vi "Actor Core.vi"(8 "error in":errorcluster, 11 "Assert Startup UI in":refnum<class "Assert Startup UI.lvclass">) -> (0 "error out":errorcluster, 3 "Actor out":refnum<class "Actor.lvclass">)   [LabVIEW 2016, in "Assert Startup UI.lvlib" / "Assert Startup UI.lvclass"]
doc: "(<B>Filename</B>: Actor Framework.lvlib:Actor.lvclass:Actor Core.vi)\n\nReceives messages to the actor, reacts to them, and initiates any error handling that may shut the actor down.\n\nDescendant classes may override this VI to append parallel tasks for the actor to complete while it handles messages. Overrides use the Call Parent Method node."
uses:
  Assert Startup UI.lvclass
  C:/Program Files (x86)/National Instruments/LabVIEW 2016/vi.lib/ActorFramework/Actor/Actor.lvclass
  D:/Work/Projects/Actor_Assert_API/Base UI Actor/Base UI Actor/Base UI Actor.lvclass
  <vilib>/ActorFramework/Actor/Actor.lvclass
  <vilib>/ActorFramework/Message Enqueuer/Message Enqueuer.lvclass
  Assert Startup UI.lvclass/Assert Startup UI.ctl
  Base UI Actor/Base UI Actor/Base UI Actor.lvclass/Base UI Actor.ctl
  <vilib>/ActorFramework/Actor/Actor.lvclass/Actor.ctl
  <vilib>/ActorFramework/Message Enqueuer/Message Enqueuer.lvclass/Message Enqueuer.ctl
  <vilib>/ActorFramework/Message Enqueuer/Init from Existing Queue.vi
  <vilib>/ActorFramework/Message Enqueuer/Enqueue.vi
  <vilib>/ActorFramework/Stop Msg/Stop Msg.lvclass
  C:/Program Files (x86)/National Instruments/LabVIEW 2016/vi.lib/ActorFramework/Message/Message.lvclass
  <vilib>/ActorFramework/Message Priority Queue/Priority Enqueue.vi
  Base UI Actor/Base UI Actor/Base UI Actor.lvclass
panel:
  in  "Add Display":bool
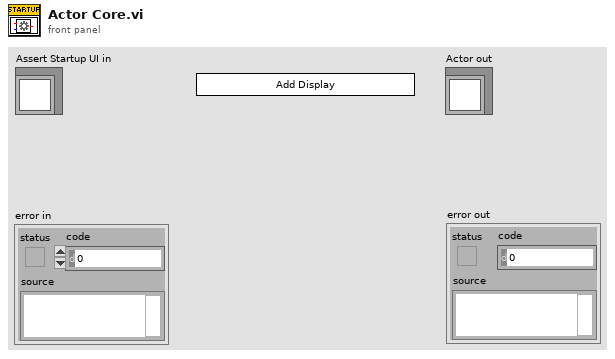
[diagram p1: front panel]
types:
  T1 = enum32{"Invalid", "Standard", "Closed", "Hidden", "Minimized", "Maximized"}
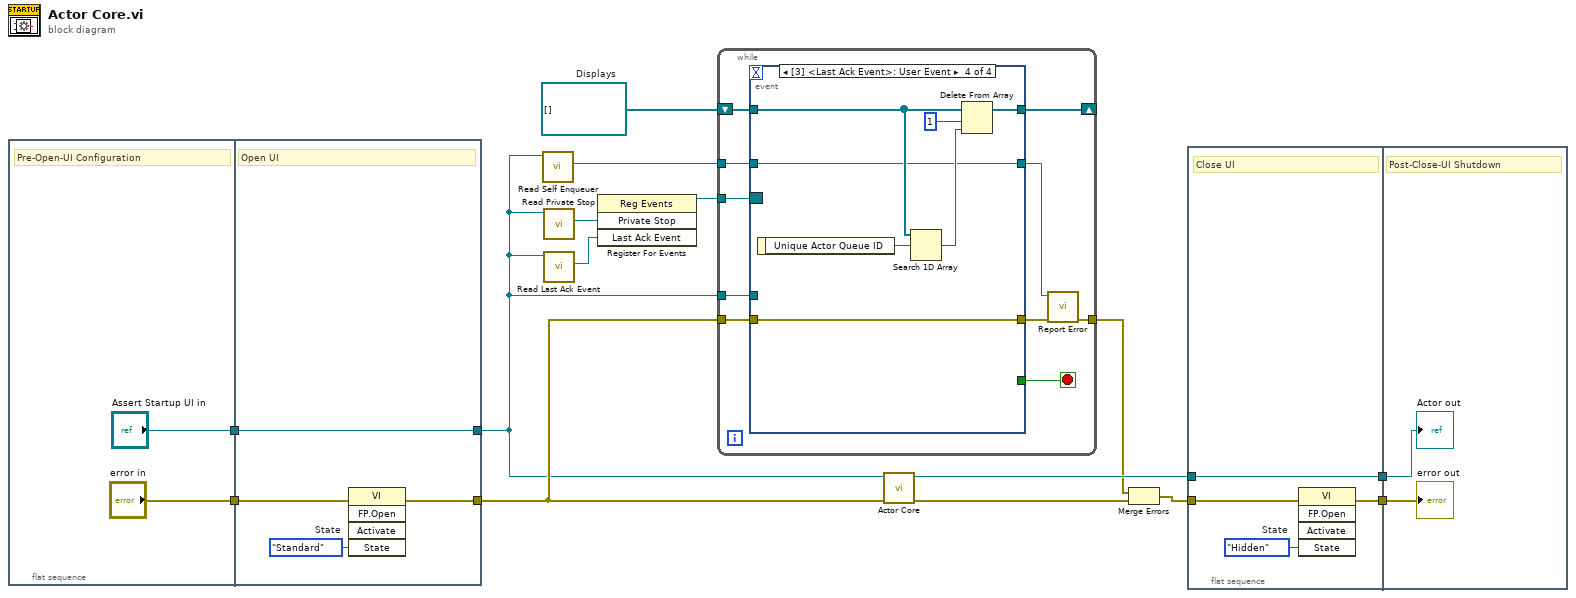
[diagram p0: block diagram]
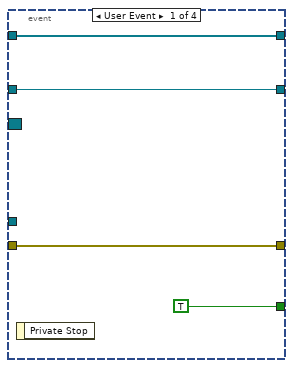
[diagram p2: hidden frame]
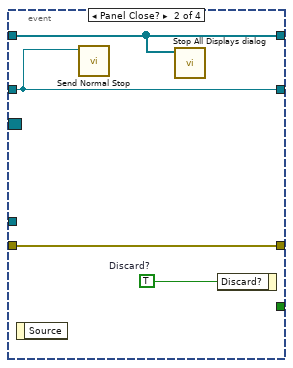
[diagram p3: hidden frame]
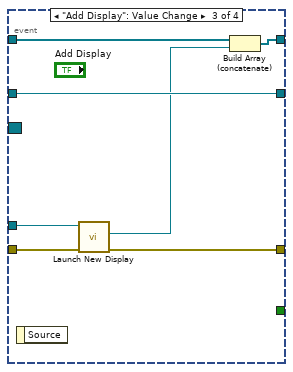
[diagram p4: hidden frame]
diagram:
  w6 = refnum<class "Message Enqueuer.lvclass">[] []  # Displays
  n1 = flat-sequence {
    tunnel: ["error in"] -> w11
    tunnel: ["Assert Startup UI in"] -> w10
    tunnel: [w20] -> w2
    tunnel: [w19] -> w5
    tunnel: w11 -> [w21]
    tunnel: w10 -> [w20]
    frame #0 {
      # "Pre-Open-UI Configuration"
    }
    frame #1 {
      w18 = T1."Standard"  # State
      # "Open UI"
      n2 = invoke class="VI" method="FP.Open"(error in=w21, "State"=w18) -> (error out=w19:errorcluster)  [unwired: 3 in, 4 out]
    }
  }
  n3 = call <vilib>:"Read Self Enqueuer.vi"("Actor"=w2) -> ("Self Enqueuer"=w7:refnum<class "Message Enqueuer.lvclass">)  [unwired: 10 in]
  n4 = call "Read Private Stop.vi"("Base UI Actor in"=w2) -> ("Private Stop"=w13:refnum<user-event>)  [unwired: 10 in]
  n5 = call "Read Last Ack Event.vi"("Assert Startup UI in"=w2) -> ("Last Ack Event"=w1:refnum<user-event>)  [unwired: 10 in]
  n6 = register-events(w13, w1) -> (reference out=w12:refnum<event-registration>)  [unwired: 2 in, 1 out]
  n7 = while {
    tunnel: w12 -> [w31]
    tunnel: w7 -> [w29]
    shift-right: [w27] -> _
    shift-left: w6 -> [w28]
    tunnel: w2 -> [w26]
    tunnel: w5 -> [w25]
    tunnel: [w23] -> w3
    stop <- w30 stop-if-true
    n8 = event shown="[3] <Last Ack Event>: User Event" {
      selector: w31 -> [_ _ _ _]
      dyn-events: _ -> [_ _ _ _]
      timeout: _ -> [_ _ _ _]
      tunnel: [TRUE _ _ _] -> w30
      tunnel: w29 -> [w32 w38 w44 w47]
      tunnel: w28 -> [w34 w37 w42 w51]
      tunnel: [w34 w37 w41 w48] -> w27
      tunnel: w26 -> [_ _ w46 _]
      tunnel: w25 -> [w33 w36 w45 w53]
      tunnel: [w32 w38 w44 w47] -> w22
      tunnel: [w33 w36 w43 w53] -> w24
      event User Event {
        n9 = event-data() -> ()  [unwired: 1 in, 1 out]
      }
      event Panel Close? {
        w39 = TRUE  # Discard?
        n10 = event-data() -> ()  [unwired: 1 in, 1 out]
        n11 = call <vilib>:"Send Normal Stop.vi"("Message Enqueuer"=w38) -> ()  [unwired: 10 in, 1 out]
        n12 = call "Stop All Displays dialog.vi"("Displays"=w37) -> ()  [unwired: 11 in]
        n13 = event-data("Discard?"=w39) -> ()  [unwired: 1 in, 1 out]
      }
      event "Add Display": Value Change {
        n14 = event-data() -> ()  [unwired: 1 in, 1 out]
        n15 = call "Launch New Display.vi"("error in (no error)"=w45, "Assert Startup UI in"=w46) -> ("error out"=w43:errorcluster, "Message Enqueuer out"=w40:refnum<class "Message Enqueuer.lvclass">)  [unwired: 8 in]
        n16 = Build Array (concatenate)(w42, w40) -> (w41:refnum<class "Message Enqueuer.lvclass">[])
      }
      event User Event {
        n17 = event-data() -> ("Unique Actor Queue ID"=w52:refnum<class "Message Enqueuer.lvclass">)  [unwired: 1 in]
        n18 = Search 1D Array(1D array=w51, element=w52) -> (index of element=w50:i32)  [unwired: 1 in]
        n19 = Delete From Array(array=w51, length=1, index=w50) -> (array with subset deleted=w48:refnum<class "Message Enqueuer.lvclass">[])  [unwired: 1 out]
      }
    }
    n20 = call "Report Error.vi"("error in (no error)"=w24, "Self Enqueuer"=w22) -> ("error out"=w23:errorcluster)  [unwired: 9 in]
  }
  n21 = call-parent "Actor Core.vi"("error in"=w5, "Actor in"=w2) -> ("error out"=w15:errorcluster, "Actor out"=w14:refnum<class "Actor.lvclass">)  [unwired: 8 in]
  n22 = Merge Errors(w3, w15) -> (w4:errorcluster)
  n23 = flat-sequence {
    tunnel: w14 -> [w57]
    tunnel: w4 -> [w56]
    tunnel: [w55] -> w9
    tunnel: [w57] -> w8
    tunnel: w9 -> [w59]
    tunnel: w8 -> [w58]
    frame #0 {
      w54 = T1."Hidden"  # State
      # "Close UI"
      n24 = invoke class="VI" method="FP.Open"(error in=w56, "State"=w54) -> (error out=w55:errorcluster)  [unwired: 3 in, 4 out]
    }
    frame #1 {
      # "Post-Close-UI Shutdown"
      "error out" <- w59
      "Actor out" <- w58
    }
  }
